vi "Read Waveform Measurement (Amplitude).vi"(0 "VISA resource name":refnum<visa-resource-name>, 1 "Maximum Time (25000ms)":u32=25000, 5 "Channel (0:Channel1)":u16(ring) items=["Channel1", "Channel2", "Channel3", "Channel4", "Math1", "Math2", "Math3", "Math3", "Reference1", "Reference2", "Reference3", "Reference4"], 7 "Function (0:Amplitude)":u16(ring) items=["Amplitude", "RMS", "Pk-Pk", "High", "Max", "Cycle RMS", "Low", "Min", "+Ovt shoot", "-Ovt shoot", "Cycle Mean", "Mean"], 11 "error in (no error)":errorcluster) -> (4 "VISA resource name out":refnum<visa-resource-name>, 6 "Measurement":dbl, 15 "error out":errorcluster)   [LabVIEW 2011, in "Tektronix 7000 Series.lvlib"]
doc: "Initiates an acquisition on the channels that you enable with the Configure Channel VI. This VI then waits for the acquisition to complete, obtains a waveform measurement on the channel you specify, and returns the measurement value."
uses:
  Tektronix 7000 Series.lvlib
  Low Level/Fetch Waveform Measurement (Amplitude).vi
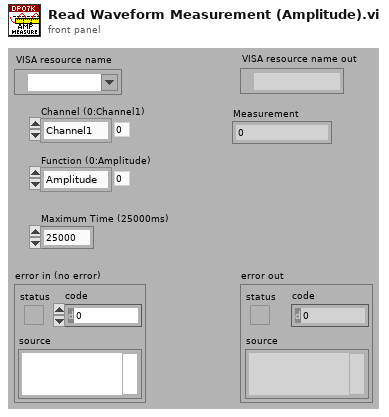
[diagram p1: front panel]
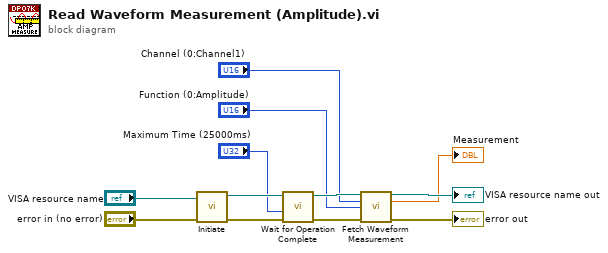
[diagram p0: block diagram]
diagram:
  n1 = call "Initiate.vi"("error in (no error)"="error in (no error)", "VISA resource name"="VISA resource name") -> ("error out"=w9:errorcluster, "VISA resource name out"=w10:refnum<visa-resource-name>)  [unwired: 8 in]
  n2 = call "Wait for Operation Complete.vi"("error in (no error)"=w9, "Maximum Time (2000ms)"="Maximum Time (25000ms)", "VISA resource name"=w10) -> ("error out"=w5:errorcluster, "VISA resource name out"=w4:refnum<visa-resource-name>)  [unwired: 7 in]
  n3 = call-poly "Fetch Waveform Measurement.vi"("VISA resource name"=w4, "Channel (0:Channel1)"="Channel (0:Channel1)", "Function (0:Amplitude)"="Function (0:Amplitude)", "error in (no error)"=w5) -> ("VISA resource name out"=→"VISA resource name out":refnum<visa-resource-name>, "Measurement"=→"Measurement":dbl, "error out"=→"error out":errorcluster)  [unwired: 9 in]
